vi "analog read.vi"(8 "error in (no error)":errorcluster, 10 "Line":string, 11 "Arduino Uno in":refnum<class "Arduino Uno.lvclass">) -> (0 "error out":errorcluster, 2 "Voltage":dbl, 3 "Arduino Uno out":refnum<class "Arduino Uno.lvclass">)   [LabVIEW 2025, in "USB IO.lvlib" / "Arduino Uno.lvclass"]
uses:
  Arduino Uno.lvclass
  Arduino Uno.lvclass/Arduino Uno.ctl
  <vilib>/MakerHub/LINX/LMH-LINX.lvlib
  <vilib>/MakerHub/LINX/Public/Peripherals/Analog/Analog Read 1 Chan.vi
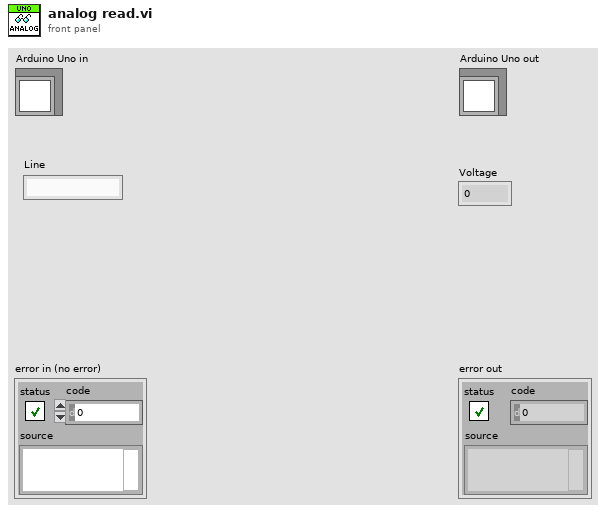
[diagram p1: front panel]
types:
  T1 = typedef "LMH-LINX.lvlib/LINX Ref.ctl" = cluster{"IO":T2, "Interface":T3, "LINX Device Config":T4}
  T2 = typedef "LMH-LINX.lvlib/Platform.ctl" = enum16{"Remote", "Local"}
  T3 = typedef "LMH-LINX.lvlib/Interface.ctl" = enum16{"Serial", "TCP"}
  T4 = typedef "LMH-LINX.lvlib/Device.lvlib/LINX Device Config.ctl" = cluster{"Interface":T3, "COM Port":refnum<visa-resource-name>, "TCP Configuration":T5, "Device Family":u8, "Device ID":u8, "Device Name":string, "TCP Ref":refnum<k5>, "Channels":T6}
  T5 = typedef "LMH-LINX.lvlib/Device.lvlib/TCP Config.ctl" = cluster{"IP Address":string, "Port":u16}
  T6 = typedef "LMH-LINX.lvlib/Channels.ctl" = cluster{"DI":u8[], "DO":u8[], "AI":u8[], "AO":u8[], "PWM":u8[], "QE":u8[], "UART":u8[], "I2C 2":u8[], "SPI":u8[], "CAN":u8[], "Servo":u8[], "AI Ref (V)":dbl, "AI Resolution (Bits)":u8, "AO Ref (V)":dbl, "AO Resolution (Bits)":u8}
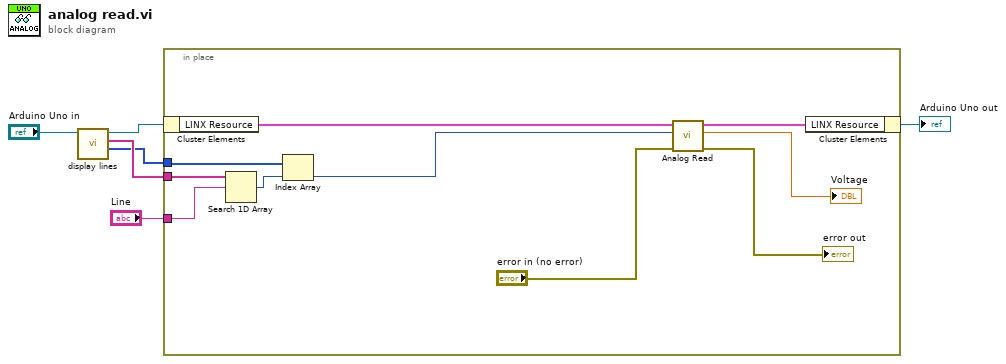
[diagram p0: block diagram]
diagram:
  n1 = call-dynamic "display lines.vi"("Arduino Uno in"="Arduino Uno in") -> ("Values"=w1:i32[], "Lines"=w2:string[], "Arduino Uno out"=w3:refnum<class "Arduino Uno.lvclass">)  [unwired: 7 in, 1 out]
  n2 = in-place {
    in-place-border: "Line" -> [w10]
    in-place-border: w2 -> [w11]
    in-place-border: w1 -> [w9]
    n3 = in-place-cluster #1(w3) -> ("LINX Resource"=w16:T1)
    n4 = Search 1D Array(1D array=w11, element=w10) -> (index of element=w8:i32)  [unwired: 1 in]
    n5 = Index Array(array=w9, index=w8) -> (element=w7:i32)
    n6 = call-poly <vilib>:"Analog Read.vi"("Error In"="error in (no error)", "Analog Channel"=w7, "LINX Resource"=w16) -> ("Error Out"=→"error out":errorcluster, "Voltage"=→"Voltage":dbl, "LINX Resource"=w15:T1)  [unwired: 5 in, 1 out]
    n7 = in-place-cluster #1("LINX Resource"=w15) -> (→"Arduino Uno out":refnum<class "Arduino Uno.lvclass">)
  }
